vi "Init Library.vi"(8 "error in (no error)":errorcluster) -> (0 "error out":errorcluster, 3 "function return":bool)   [LabVIEW 2015, in "XGL_DPP.lvlib"]
doc: "EXTERN DECLSPEC bool CALL_CONV InitLibrary(void);"
uses:
  XGL_DPP.lvlib
  XGL_DPP.dll
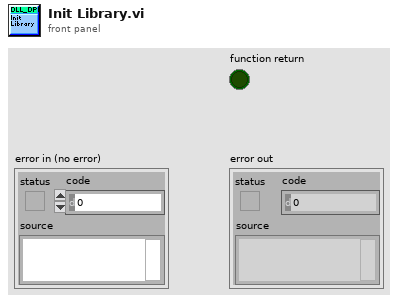
[diagram p1: front panel]
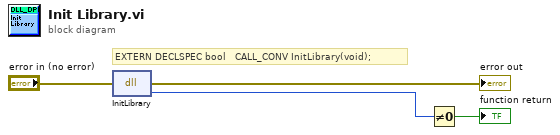
[diagram p0: block diagram]
diagram:
  # "EXTERN DECLSPEC bool   CALL_CONV InitLibrary(void);"
  n1 = dll-call lib="D:/Users/XRF/Desktop/Dante_acquire4/libs/Dante/XGL_DPP.dll" fn="InitLibrary"(error in="error in (no error)") -> (error out=→"error out":errorcluster, "return type"=w3:u8)  [unwired: 2 in, 1 out]
  n2 = Not Equal To 0?(x=w3) -> (x != 0?=→"function return":bool)
